vi "USB2XXX_LINEX_MasterSchTest.vi"() -> ()   [LabVIEW 2010]
panel:
  in  "stop 2":bool
  out "设置调度表成功？":bool
  in  "pInMsg 3":T1={"Timestamp"=50, "MsgType"=2, "CheckType"=0, "DataLen"=0, "Sync"=85, "PID"=3, "Data[0]"=0, "Data[1]"=0, "Data[2]"=0, "Data[3]"=0, "Data[4]"=0, "Data[5]"=0, "Data[6]"=0, "Data[7]"=0, "Check"=0, "Reserve"=0, "Reserve"=0} {"Sync" format="%x"; "PID" format="%x"; "Data[0]" format="%x"; "Data[1]" format="%x"; "Data[2]" format="%x"; "Data[3]" format="%x"; "Data[4]" format="%x"; "Data[5]" format="%x"; "Data[6]" format="%x"; "Data[7]" format="%x"; "Check" format="%x"; "Reserve" format="%x"; "Reserve" format="%x"}
  in  "pInMsg 2":T1={"Timestamp"=50, "MsgType"=2, "CheckType"=0, "DataLen"=8, "Sync"=85, "PID"=2, "Data[0]"=17, "Data[1]"=34, "Data[2]"=51, "Data[3]"=68, "Data[4]"=85, "Data[5]"=102, "Data[6]"=119, "Data[7]"=136, "Check"=0, "Reserve"=0, "Reserve"=0} {"Sync" format="%x"; "PID" format="%x"; "Data[0]" format="%x"; "Data[1]" format="%x"; "Data[2]" format="%x"; "Data[3]" format="%x"; "Data[4]" format="%x"; "Data[5]" format="%x"; "Data[6]" format="%x"; "Data[7]" format="%x"; "Check" format="%x"; "Reserve" format="%x"; "Reserve" format="%x"}
  out "pOutMsg":T2(array[cluster]) {"Sync" format="%x"; "PID" format="%x"; "Data[0]" format="%x"; "Data[1]" format="%x"; "Data[2]" format="%x"; "Data[3]" format="%x"; "Data[4]" format="%x"; "Data[5]" format="%x"; "Data[6]" format="%x"; "Data[7]" format="%x"; "Check" format="%x"}
  in  "pInMsg":T1={"Timestamp"=50, "MsgType"=1, "CheckType"=0, "DataLen"=8, "Sync"=85, "PID"=1, "Data[0]"=1, "Data[1]"=2, "Data[2]"=3, "Data[3]"=4, "Data[4]"=5, "Data[5]"=6, "Data[6]"=7, "Data[7]"=8, "Check"=0, "Reserve"=0, "Reserve"=0} {"Sync" format="%x"; "PID" format="%x"; "Data[0]" format="%x"; "Data[1]" format="%x"; "Data[2]" format="%x"; "Data[3]" format="%x"; "Data[4]" format="%x"; "Data[5]" format="%x"; "Data[6]" format="%x"; "Data[7]" format="%x"; "Check" format="%x"; "Reserve" format="%x"; "Reserve" format="%x"}
  out "function return":i32
  in  "BaudRate":u32=19200
  in  "Channel Index":u8(ring) items=["LIN1", "LIN2"]
  in  "Device Index":i32(ring) items=["0", "1", "2", "3", "4", "5"]
  # "运行程序后，适配器自动发送界面中的3帧数据，间隔时间为50ms，同时自动读取调度表，可以获取调度表运行数据"
  # "波特率一定要设置，否则程序可能出错"
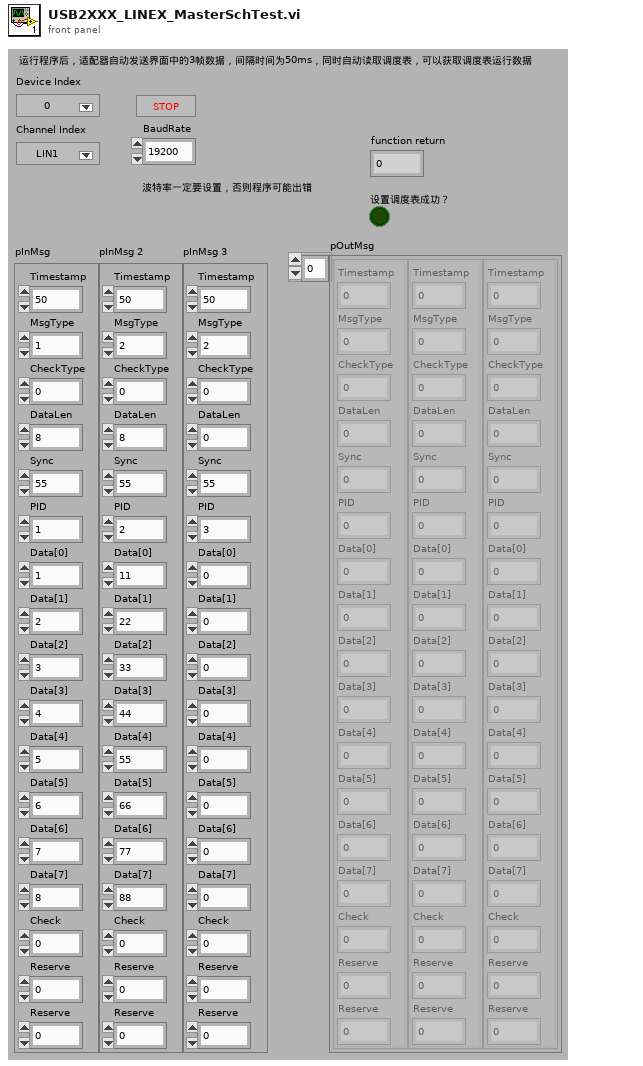
[diagram p1: front panel]
types:
  T1 = cluster{"Timestamp":u32, "MsgType":u8, "CheckType":u8, "DataLen":u8, "Sync":u8, "PID":u8, "Data[0]":u8, "Data[1]":u8, "Data[2]":u8, "Data[3]":u8, "Data[4]":u8, "Data[5]":u8, "Data[6]":u8, "Data[7]":u8, "Check":u8, "Reserve":u8, "Reserve":u8}
  T2 = cluster{"Timestamp":u32, "MsgType":u8, "CheckType":u8, "DataLen":u8, "Sync":u8, "PID":u8, "Data[0]":u8, "Data[1]":u8, "Data[2]":u8, "Data[3]":u8, "Data[4]":u8, "Data[5]":u8, "Data[6]":u8, "Data[7]":u8, "Check":u8, "Reserve":u8, "Reserve":u8}[]
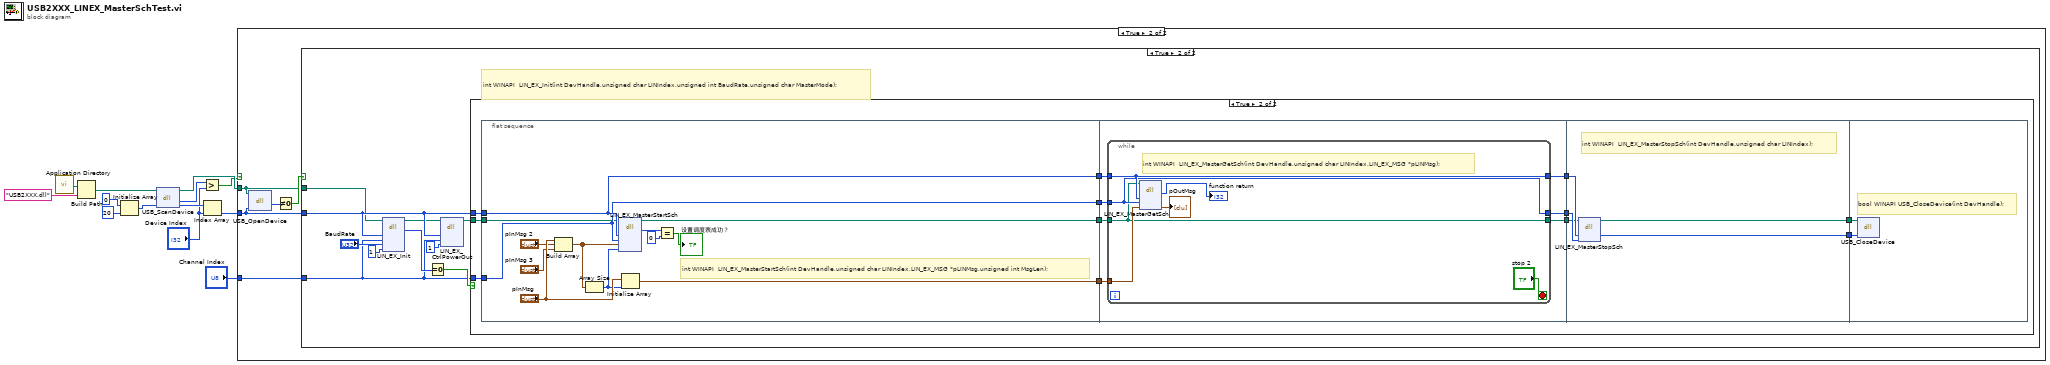
[diagram p0: block diagram]
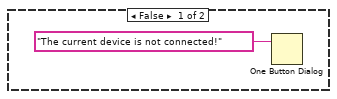
[diagram p2: hidden frame]
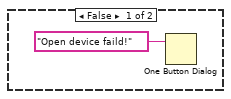
[diagram p3: hidden frame]
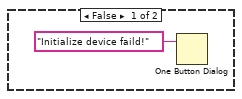
[diagram p4: hidden frame]
diagram:
  n1 = call <vilib>:"Application Directory.vi"() -> ("Application Directory"=w6:path)
  n2 = Build Path(base path=w6, name or relative path="USB2XXX.dll") -> (appended path=w5:path)
  n3 = Initialize Array(0, 20 ("dimension size")) -> (w10:i32[])
  n4 = dll-call lib="E:/OtherWork/STM32/USB2XXX_Example/trunk/Labview/PublicFiles/USB2XXX.dll" fn="USB_ScanDevice"(path in=w5, "pDevNum"=w10) -> (path out=w9:path, "return type"=w3:i32, "pDevNum"=w13:i32[])  [unwired: 2 in, 1 out]
  n5 = Greater?(x=w3, y="Device Index") -> (0:w4:bool)
  n6 = Index Array(array=w13, index="Device Index") -> (element=w8:i32)
  n7 = case shown="True" w4 {
    tunnel: w9 -> [_ w16]
    tunnel: w8 -> [_ w17]
    tunnel: "Channel Index" -> [_ w15]
    frame False {
      n8 = One Button Dialog(message="The current device is not connected!") -> ()  [unwired: 1 in, 1 out]
    }
    frame True {
      n9 = dll-call lib="E:/OtherWork/STM32/USB2XXX_Example/trunk/Labview/PublicFiles/USB2XXX.dll" fn="USB_OpenDevice"(path in=w16, "DevIndex"=w17) -> ("return type"=w19:u8)  [unwired: 3 in, 2 out]
      n10 = Not Equal To 0?(x=w19) -> (x != 0?=w18:bool)
      n11 = case shown="True" w18 {
        tunnel: w17 -> [_ w26]
        tunnel: w16 -> [_ w23]
        tunnel: w15 -> [_ w25]
        frame False {
          n12 = One Button Dialog(message="Open device faild!") -> ()  [unwired: 1 in, 1 out]
        }
        frame True {
          # "int WINAPI  LIN_EX_Init(int DevHandle,unsigned char LINIndex,unsigned int BaudRate,unsigned char MasterMode);"
          n13 = dll-call lib="E:/OtherWork/STM32/USB2XXX_Example/trunk/Labview/PublicFiles/USB2XXX.dll" fn="LIN_EX_Init"(path in=w23, "DevHandle"=w26, "LINIndex"=w25, "BaudRate"="BaudRate", "MasterMode"=u8 1) -> (path out=w22:path, "return type"=w30:i32)  [unwired: 6 in, 1 out]
          n14 = Equal To 0?(x=w30) -> (x = 0?=w29:bool)
          n15 = dll-call lib="E:/Projects/USB2XXX/trunk/USB2XXX/USB2XXX/vs2010/Release/USB2XXX.*" fn="LIN_EX_CtrlPowerOut"(path in=w22, "DevHandle"=w26, "LINIndex"=w25, "VbatValue"=u8 1) -> (path out=w21:path)  [unwired: 6 in, 1 out]
          n16 = case shown="True" w29 {
            tunnel: w26 -> [_ w43]
            tunnel: w25 -> [_ w42]
            tunnel: w21 -> [_ w38]
            frame False {
              n17 = One Button Dialog(message="Initialize device faild!") -> ()  [unwired: 1 in, 1 out]
            }
            frame True {
              n18 = flat-sequence {
                tunnel: w43 -> [w47]
                tunnel: w42 -> [w46]
                tunnel: [w48] -> w41
                tunnel: [w47] -> w40
                tunnel: [w46] -> w39
                tunnel: w38 -> [w45]
                tunnel: [w44] -> w37
                tunnel: w41 -> [w63]
                tunnel: w40 -> [w62]
                tunnel: w39 -> [w61]
                tunnel: w37 -> [w60]
                tunnel: [w59] -> w36
                tunnel: [w58] -> w35
                tunnel: [w57] -> w34
                tunnel: w36 -> [w75]
                tunnel: w35 -> [w74]
                tunnel: w34 -> [w73]
                tunnel: [w72] -> w33
                tunnel: [w71] -> w32
                tunnel: w33 -> [w77]
                tunnel: w32 -> [w76]
                frame #0 {
                  # "int WINAPI  LIN_EX_MasterStartSch(int DevHandle,unsigned char LINIndex,LIN_EX_MSG *pLINMsg,unsigned int MsgLen);"
                  n19 = Build Array("pInMsg", "pInMsg 2", "pInMsg 3") -> (w50:T2)
                  n20 = Array Size(array=w50) -> (size(s)=w49:i32)
                  n21 = dll-call lib="E:/OtherWork/STM32/USB2XXX_Example/trunk/Labview/PublicFiles/USB2XXX.*" fn="LIN_EX_MasterStartSch"(path in=w45, "DevHandle"=w47, "LINIndex"=w46, "pLINMsg"=w50, "MsgLen"=w49) -> (path out=w44:path, "return type"=w54:i32)  [unwired: 6 in, 1 out]
                  n22 = Initialize Array("pInMsg", w49) -> (w48:T2)
                  n23 = Equal?(x=w54, y=0) -> (x = y?=→"设置调度表成功？":bool)
                }
                frame #1 {
                  n24 = while {
                    tunnel: w63 -> [w68]
                    tunnel: w62 -> [w66]
                    tunnel: w61 -> [w65]
                    tunnel: w60 -> [w64]
                    tunnel: [w66] -> w59
                    tunnel: [w65] -> w58
                    tunnel: [w64] -> w57
                    stop <- "stop 2" stop-if-true
                    # "int WINAPI  LIN_EX_MasterGetSch(int DevHandle,unsigned char LINIndex,LIN_EX_MSG *pLINMsg);"
                    n25 = dll-call lib="E:/OtherWork/STM32/USB2XXX_Example/trunk/Labview/PublicFiles/USB2XXX.*" fn="LIN_EX_MasterGetSch"(path in=w64, "DevHandle"=w66, "LINIndex"=w65, "pLINMsg"=w68) -> ("return type"=→"function return":i32, "pLINMsg"=→"pOutMsg":T2)  [unwired: 4 in, 2 out]
                  }
                }
                frame #2 {
                  # "int WINAPI  LIN_EX_MasterStopSch(int DevHandle,unsigned char LINIndex);"
                  n26 = dll-call lib="E:/OtherWork/STM32/USB2XXX_Example/trunk/Labview/PublicFiles/USB2XXX.*" fn="LIN_EX_MasterStopSch"(path in=w73, "DevHandle"=w75, "LINIndex"=w74) -> (path out=w71:path, "DevHandle"=w72:i32)  [unwired: 4 in, 1 out]
                }
                frame #3 {
                  # "bool WINAPI USB_CloseDevice(int DevHandle);"
                  n27 = dll-call lib="E:/Projects/USB2XXX/trunk/USB2XXX/USB2XXX/vs2010/Release/USB2XXX.*" fn="USB_CloseDevice"(path in=w76, "DevHandle"=w77) -> ()  [unwired: 4 in, 2 out]
                }
              }
            }
          }
        }
      }
    }
  }
